vi "Enqueue Data.vi"(2 "error in (no error)":errorcluster, 4 "Message Data":variant, 5 "data info":string) -> (0 "error out":errorcluster, 1 "created new?":bool)   [LabVIEW 2016, in "Message Queue.lvlib"]
uses:
  Message Queue.lvlib
  Data queue name (constant).ctl
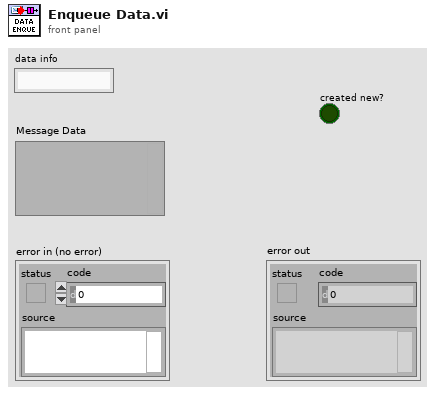
[diagram p1: front panel]
types:
  T1 = typedef "Message Queue.lvlib/Data queue name (constant).ctl" = string
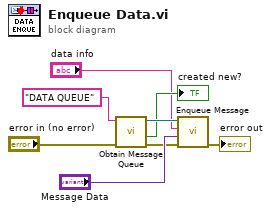
[diagram p0: block diagram]
diagram:
  n1 = call "Obtain Message Queue.vi"("error in (no error)"="error in (no error)", "name (unnamed)"=T1 "DATA QUEUE") -> ("error out"=w5:errorcluster, "created new?"=→"created new?":bool, "Message Queue"=w7:refnum<queue>)  [unwired: 7 in]
  n2 = call "Enqueue Message.vi"("error in (no error)"=w5, "Message Data"="Message Data", "Message"="data info", "Message Queue"=w7) -> ("error out"=→"error out":errorcluster)  [unwired: 6 in, 1 out]
